vi "日志、报警信息存储 (子VI).vi"() -> ()   [LabVIEW 2016, in "超标留样集成.lvlib" / "德润DR803F超标留样.lvlib"]
uses:
  <vilib>/ptbypt/NI_PtbyPt.lvlib
panel:
  out "仪器状态":T1 {"门状态" items=["关闭", "打开"]; "采样模式" items=["定时留样"=1, "时间等比"=2, "同步留样"=3, "外控留样"=4, "超标留样"=5]; "工作进程" items=["清洗管路初始化", "采样瓶位置初始化", "采样瓶排空", "清洗管下降", "采样瓶清洗", "清洗管上升", "外置泵延时", "管路润洗", "进样1", "进样2", "排空管路", "采样瓶位置调整", "待机"]; "仪器时间" format="%<%Y/%m/%d %H:%M:%S>T"; "工作状态" items=["停止", "运行"]}
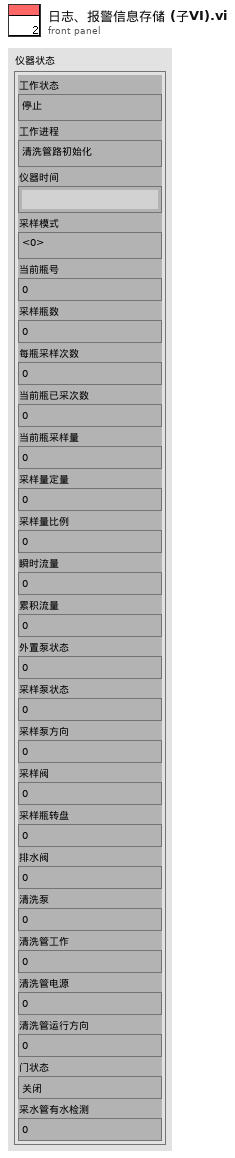
[diagram p1: front panel]
types:
  T1 = cluster{"工作状态":u16, "工作进程":u16, "仪器时间":timestamp, "采样模式":u16, "当前瓶号":dbl, "采样瓶数":dbl, "每瓶采样次数":dbl, "当前瓶已采次数":dbl, "当前瓶采样量":dbl, "采样量定量":dbl, "采样量比例":dbl, "瞬时流量":dbl, "累积流量":dbl, "外置泵状态":dbl, "采样泵状态":dbl, "采样泵方向":dbl, "采样阀":dbl, "采样瓶转盘":dbl, "排水阀":dbl, "清洗泵":dbl, "清洗管工作":dbl, "清洗管电源":dbl, "清洗管运行方向":dbl, "门状态":u16, "采水管有水检测":dbl}
  T2 = cluster{"时间标识":timestamp, "设备":string, "日志信息":string}
  T3 = cluster{"时间标识":timestamp, "设备":string, "日志信息":string, "流程参数":string}
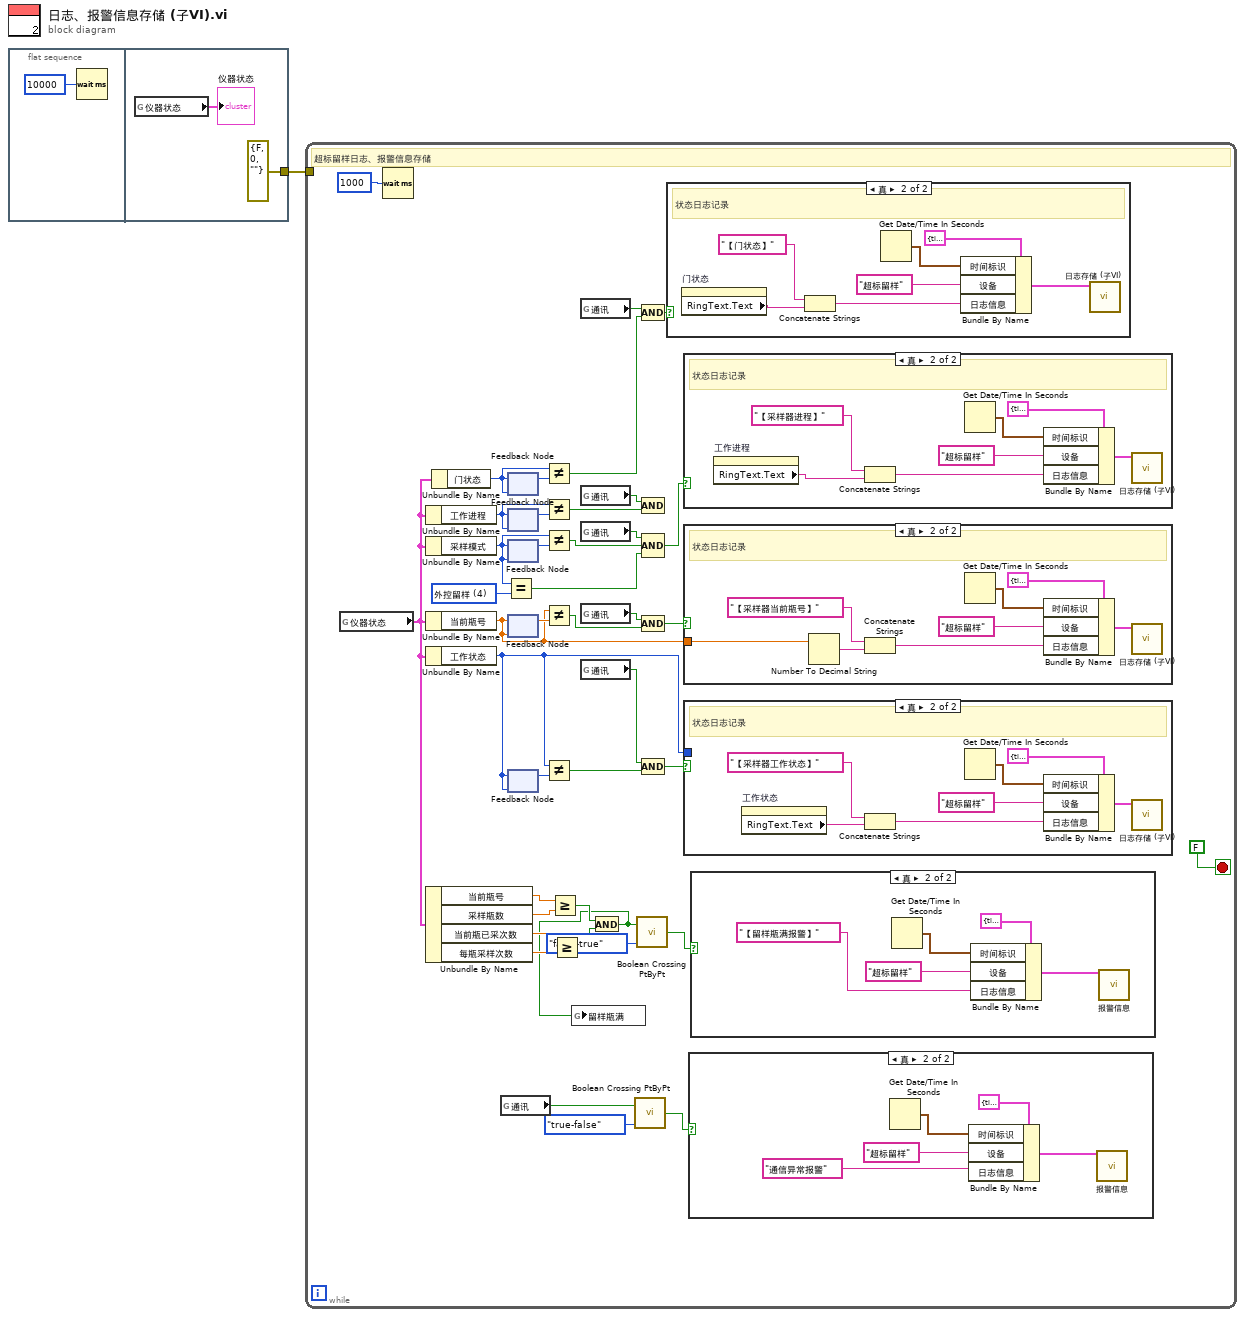
[diagram p0: block diagram]
diagram:
  n1 = flat-sequence {
    tunnel: [errorcluster {"status"=FALSE, "code"=0, "source"=""} ("错误常量")] -> w1
    frame #0 {
      n2 = Wait (ms)(milliseconds to wait=u32 10000 ("等待时间（毫秒）")) -> ()  [unwired: 1 out]
    }
    frame #1 {
      n3 = global read "超标留样全局.vi" "仪器状态"() -> (→"仪器状态":T1)
    }
  }
  n4 = while {
    tunnel: w1 -> [_]
    stop <- FALSE stop-if-true
    w19 = u16 4 items=["定时留样"=1, "时间等比"=2, "同步留样"=3, "外控留样"=4, "超标留样"=5] ("采样模式")
    # "超标留样日志、报警信息存储"
    n5 = global read "超标留样全局.vi" "仪器状态"() -> (w17:T1)
    n6 = Wait (ms)(milliseconds to wait=u32 1000 ("等待时间（毫秒）")) -> ()  [unwired: 1 out]
    n7 = Unbundle By Name(w17) -> ("工作进程"=w43:u16)
    n8 = Unbundle By Name(w17) -> ("采样模式"=w35:u16)
    n9 = Unbundle By Name(w17) -> ("当前瓶号"=w40:dbl)
    n10 = Unbundle By Name(w17) -> ("工作状态"=w39:u16)
    n11 = Unbundle By Name(w17) -> ("当前瓶号"=w14:dbl, "采样瓶数"=w13:dbl, "当前瓶已采次数"=w12:dbl, "每瓶采样次数"=w11:dbl)
    n12 = Unbundle By Name(w17) -> ("门状态"=w36:u16)
    n13 = global read "超标留样全局.vi" "通讯"() -> (w6:bool)
    n14 = Equal?(x=w35, y=w19) -> (x = y?=w21:bool)
    n15 = feedback #1(w36) -> (w37:u16)
    n16 = feedback-in #1(w36) -> ()
    n17 = feedback #2(w43) -> (w42:u16)
    n18 = feedback-in #2(w43) -> ()
    n19 = feedback #3(w35) -> (w34:u16)
    n20 = feedback-in #3(w35) -> ()
    n21 = feedback #4(w40) -> (w41:dbl)
    n22 = feedback-in #4(w40) -> ()
    n23 = feedback #5(w39) -> (w38:u16)
    n24 = feedback-in #5(w39) -> ()
    n25 = Not Equal?(x=w36, y=w37) -> (x != y?=w31:bool)
    n26 = Not Equal?(x=w43, y=w42) -> (x != y?=w29:bool)
    n27 = Not Equal?(x=w35, y=w34) -> (x != y?=w20:bool)
    n28 = Not Equal?(x=w40, y=w41) -> (x != y?=w26:bool)
    n29 = Not Equal?(x=w39, y=w38) -> (x != y?=w24:bool)
    n30 = Greater Or Equal?(x=w14, y=w13) -> (x >= y?=w16:bool)
    n31 = Greater Or Equal?(x=w12, y=w11) -> (x >= y?=w15:bool)
    n32 = global read "超标留样全局.vi" "通讯"() -> (w33:bool)
    n33 = global read "超标留样全局.vi" "通讯"() -> (w30:bool)
    n34 = global read "超标留样全局.vi" "通讯"() -> (w22:bool)
    n35 = global read "超标留样全局.vi" "通讯"() -> (w28:bool)
    n36 = global read "超标留样全局.vi" "通讯"() -> (w25:bool)
    n37 = And(x=w16, y=w15) -> (x .and. y?=w5:bool)
    n38 = global write "超标留样全局.vi" "留样瓶满"(w5) -> ()
    n39 = call <vilib>:"Boolean Crossing PtByPt.vi"("direction"=enum16{"either", "false-true", "true-false"}."true-false", "input"=w6) -> ("crossing"=w8:bool)  [unwired: 1 in]
    n40 = call <vilib>:"Boolean Crossing PtByPt.vi"("direction"=enum16{"either", "false-true", "true-false"}."false-true", "input"=w5) -> ("crossing"=w9:bool)  [unwired: 1 in]
    n41 = Compound Arithmetic op=AND ("复合运算")(w33, w31) -> (w32:bool)
    n42 = Compound Arithmetic op=AND ("复合运算")(w30, w29) -> ()  [unwired: 1 out]
    n43 = Compound Arithmetic op=AND ("复合运算")(w22, w20, w21) -> (w18:bool)
    n44 = Compound Arithmetic op=AND ("复合运算")(w28, w26) -> (w27:bool)
    n45 = Compound Arithmetic op=AND ("复合运算")(w25, w24) -> (w23:bool)
    n46 = case shown="真" w32 {
      frame False {
      }
      frame True {
        # "状态日志记录"
        n47 = property on="门状态" class="Ring (严格)"() -> ("RingText.Text"=w56:string)  [unwired: 2 in, 2 out]
        n48 = Concatenate Strings("【门状态】" ("日志信息"), w56) -> (w62:string)
        n49 = Get Date/Time In Seconds() -> (seconds since 1Jan1904=w59:timestamp)
        n50 = Bundle By Name(cluster=T3 {"时间标识"=timestamp(0 s since 1904-01-01), "设备"="", "日志信息"="", "流程参数"=""} ("data in"), "时间标识"=w59, "设备"="超标留样", "日志信息"=w62) -> (w58:T3)
        n51 = call "日志存储 (子VI).vi"("data in"=w58) -> ()  [unwired: 11 in]
      }
    }
    n52 = case shown="真" w18 {
      frame False {
      }
      frame True {
        # "状态日志记录"
        n53 = property on="工作进程" class="Ring (严格)"() -> ("RingText.Text"=w78:string)  [unwired: 2 in, 2 out]
        n54 = Concatenate Strings("【采样器进程】" ("日志信息"), w78) -> (w84:string)
        n55 = Get Date/Time In Seconds() -> (seconds since 1Jan1904=w81:timestamp)
        n56 = Bundle By Name(cluster=T3 {"时间标识"=timestamp(0 s since 1904-01-01), "设备"="", "日志信息"="", "流程参数"=""} ("data in"), "时间标识"=w81, "设备"="超标留样", "日志信息"=w84) -> (w80:T3)
        n57 = call "日志存储 (子VI).vi"("data in"=w80) -> ()  [unwired: 11 in]
      }
    }
    n58 = case shown="真" w27 {
      tunnel: w40 -> [_ w71]
      frame False {
      }
      frame True {
        # "状态日志记录"
        n59 = Number To Decimal String(number=w71) -> (decimal integer string=w70:string)  [unwired: 1 in]
        n60 = Concatenate Strings("【采样器当前瓶号】" ("日志信息"), w70) -> (w77:string)
        n61 = Get Date/Time In Seconds() -> (seconds since 1Jan1904=w74:timestamp)
        n62 = Bundle By Name(cluster=T3 {"时间标识"=timestamp(0 s since 1904-01-01), "设备"="", "日志信息"="", "流程参数"=""} ("data in"), "时间标识"=w74, "设备"="超标留样", "日志信息"=w77) -> (w73:T3)
        n63 = call "日志存储 (子VI).vi"("data in"=w73) -> ()  [unwired: 11 in]
      }
    }
    n64 = case shown="真" w23 {
      tunnel: w39 -> [_ _]
      frame False {
      }
      frame True {
        # "状态日志记录"
        n65 = property on="工作状态" class="Ring (严格)"() -> ("RingText.Text"=w63:string)  [unwired: 2 in, 2 out]
        n66 = Concatenate Strings("【采样器工作状态】" ("日志信息"), w63) -> (w69:string)
        n67 = Get Date/Time In Seconds() -> (seconds since 1Jan1904=w66:timestamp)
        n68 = Bundle By Name(cluster=T3 {"时间标识"=timestamp(0 s since 1904-01-01), "设备"="", "日志信息"="", "流程参数"=""} ("data in"), "时间标识"=w66, "设备"="超标留样", "日志信息"=w69) -> (w65:T3)
        n69 = call "日志存储 (子VI).vi"("data in"=w65) -> ()  [unwired: 11 in]
      }
    }
    n70 = case shown="真" w8 {
      frame False {
      }
      frame True {
        n71 = Get Date/Time In Seconds() -> (seconds since 1Jan1904=w49:timestamp)
        n72 = Bundle By Name(cluster=T2 {"时间标识"=timestamp(0 s since 1904-01-01), "设备"="", "日志信息"=""} ("data in"), "时间标识"=w49, "设备"="超标留样", "日志信息"="通信异常报警") -> (w47:T2)
        n73 = call "报警信息.vi"("data in"=w47) -> ()  [unwired: 10 in, 1 out]
      }
    }
    n74 = case shown="真" w9 {
      frame False {
      }
      frame True {
        n75 = Get Date/Time In Seconds() -> (seconds since 1Jan1904=w54:timestamp)
        n76 = Bundle By Name(cluster=T2 {"时间标识"=timestamp(0 s since 1904-01-01), "设备"="", "日志信息"=""} ("data in"), "时间标识"=w54, "设备"="超标留样", "日志信息"="【留样瓶满报警】") -> (w51:T2)
        n77 = call "报警信息.vi"("data in"=w51) -> ()  [unwired: 10 in, 1 out]
      }
    }
  }
